vi "SIRRect.vi"(8 "P":cluster{"x":dbl, "y":dbl, "z":dbl}={"x"=1.0, "y"=-5.0, "z"=1.0} {"x" format="%.2f"; "z" format="%.2f"; "y" format="%.2f"}, 9 "Variables":T1={"sound spd (cm/s)"=150000, "time step (s)"=1e-09} {"time step (s)" format="%.2e"}, 11 "strip":cluster{"Radius":dbl, "h":dbl, "a":dbl}={"Radius"=10.0, "h"=3.0, "a"=5.0} {"Radius" format="%.2f"; "a" format="%.2f"; "h" format="%.2f"}) -> (1 "lower":dbl[](graph), 2 "upper":dbl[](graph), 3 "h rect":dbl[](graph), 4 "delay out":i32)   [LabVIEW 2022 SP3]
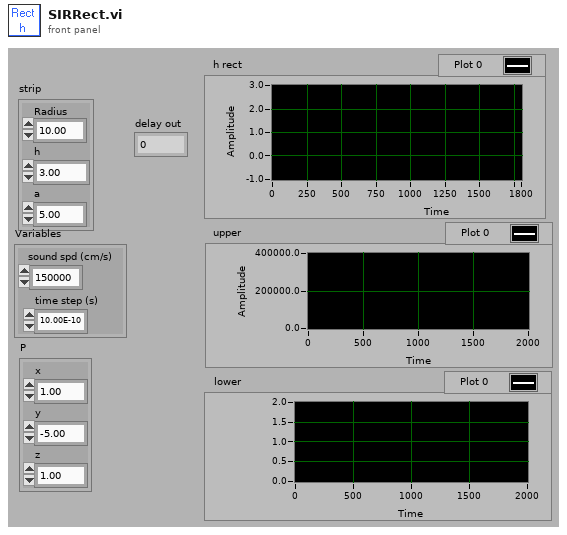
[diagram p1: front panel]
types:
  T1 = cluster{"sound spd (cm/s)":i32, "time step (s)":sgl}
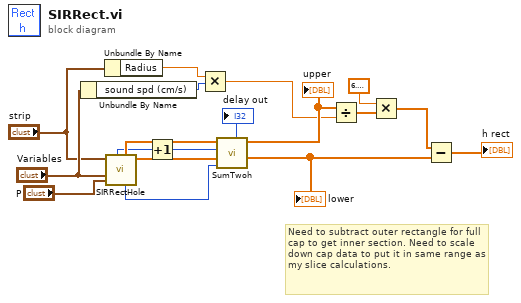
[diagram p0: block diagram]
diagram:
  # "Need to subtract outer rectangle for full cap to get inner section. Need to scale down cap data to put it in same range as my slice calculations."
  n1 = Unbundle By Name("Variables") -> ("sound spd (cm/s)"=w6:i32)
  n2 = Unbundle By Name("strip") -> ("Radius"=w7:dbl)
  n3 = call "SIRRectHole.vi"("P"="P", "Variables"="Variables", "strip"="strip") -> ("h rect"=w16:dbl[], "delay out"=w17:i32, "h cap"=w15:dbl[], "cap delay pts"=w14:i32)  [unwired: 5 out]
  n4 = Increment(x=w14) -> (x+1=w1:i32)
  n5 = Multiply(x=w7, y=w6) -> (x*y=w5:dbl)
  n6 = call "SumTwoh.vi"("h1"=w15, "delay1"=w1, "h2"=w16, "delay2"=w17) -> ("delay out"=→"delay out":i32, "upper"=w10:dbl[], "lower"=w12:dbl[])  [unwired: 2 out]
  "upper" <- w10
  "lower" <- w12
  n7 = Divide(x=w10, y=w5) -> (x/y=w4:dbl[])
  n8 = Multiply(x=6.283185307179586, y=w4) -> (x*y=w3:dbl[])
  n9 = Subtract(x=w3, y=w12) -> (x-y=→"h rect":dbl[])
